vi "ActionVIOnDelete.vi"(6 "All deleted Refs":T1[](array[typedef]) format="%.0x", 8 "error in (no error)":errorcluster, 11 "Item Ref in":T1 format="%.0x") -> (0 "error out":errorcluster, 3 "Item Ref out":T1 format="%.0x")   [LabVIEW 2015, in "UDP-Custom-Device System Explorer.lvlib"]
uses:
  UDP-Custom-Device System Explorer.lvlib
  <vilib>/NI Veristand/Custom Device API/Custom Device Item Ref.ctl
  Shared/Constants.vi
  <vilib>/NI Veristand/Custom Device Tools/Custom Device Utility Library/NI VeriStand - Search for Item by GUID.vi
  <vilib>/NI VeriStand/Custom Device Tools/Custom Device Utility Library/Custom Device Utility Library.lvlib
  Shared/UDP-Custom-Device Shared.lvlib
  <vilib>/NI VeriStand/Custom Device API/Custom Device API.lvlib
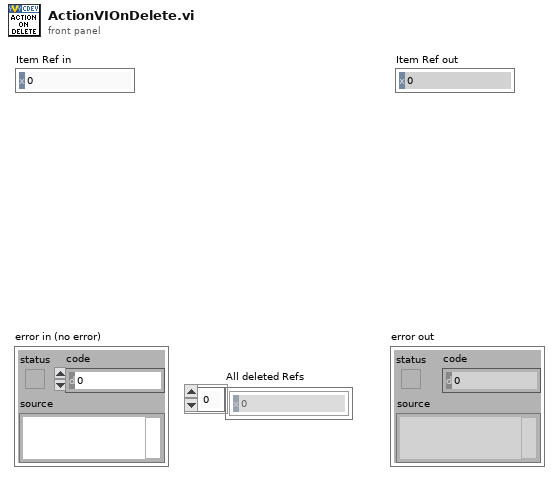
[diagram p1: front panel]
types:
  T1 = typedef "Custom Device API.lvlib/Custom Device Item Ref.ctl" = u64
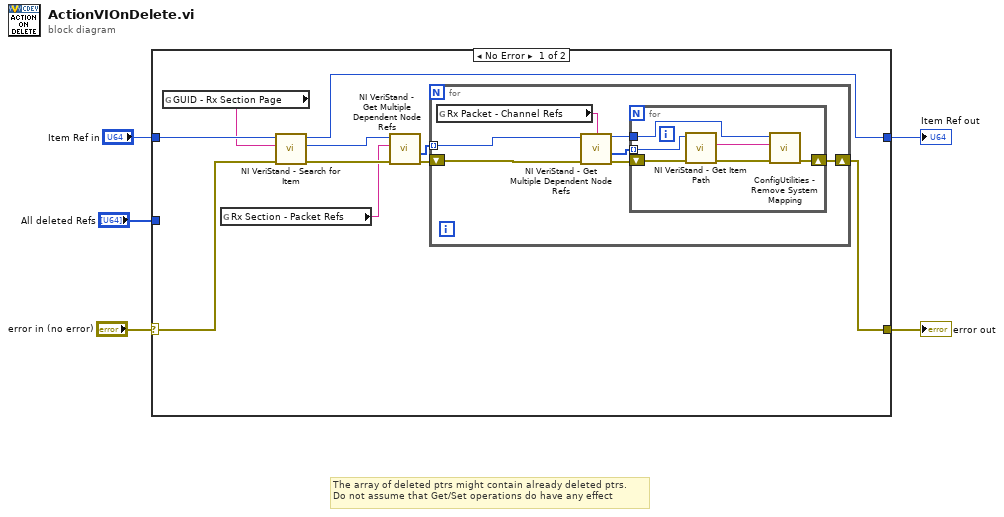
[diagram p0: block diagram]
diagram:
  # "The array of deleted ptrs might contain already deleted ptrs.\nDo not assume that Get/Set operations do have any effect"
  n1 = case shown="No Error" "error in (no error)" {
    selector: "error in (no error)" -> [w14 w30]
    tunnel: [w13 w30] -> w4
    tunnel: "Item Ref in" -> [w15 w29]
    tunnel: [w11 w29] -> w2
    tunnel: "All deleted Refs" -> [_ _]
    frame No Error {
      n2 = global read "Constants.vi" "GUID - Rx Section Page"() -> (w12:string)
      n3 = global read "Constants.vi" "Rx Section - Packet Refs"() -> (w8:string)
      n4 = call-poly <vilib>:"NI VeriStand - Search for Item.vi"("error in"=w14, "Item GUID"=w12, "Section Ref in"=w15) -> ("error out"=w10:errorcluster, "Item Ref"=w9:T1, "Section Ref out"=w11:T1)  [unwired: 5 in, 1 out]
      n5 = call <vilib>:"NI VeriStand - Get Multiple Dependent Node Refs.vi"("error in (no error)"=w10, "Base Property Name"=w8, "Item Ref in"=w9) -> ("error out"=w7:errorcluster, "Dependent Node Refs"=w6:T1[])  [unwired: 6 in, 1 out]
      n6 = for {
        tunnel: w6 -> [w16] mode=indexing
        shift-right: [w19] -> w13
        shift-left: w7 -> [w22]
        n7 = global read "Constants.vi" "Rx Packet - Channel Refs"() -> (w21:string)
        n8 = call <vilib>:"NI VeriStand - Get Multiple Dependent Node Refs.vi"("error in (no error)"=w22, "Base Property Name"=w21, "Item Ref in"=w16) -> ("error out"=w20:errorcluster, "Dependent Node Refs"=w17:T1[], "Item Ref out"=w18:T1)  [unwired: 6 in]
        n9 = for {
          shift-right: [w28] -> w19
          shift-left: w20 -> [w25]
          tunnel: w18 -> [w23]
          tunnel: w17 -> [w24] mode=indexing
          n10 = call <vilib>:"NI VeriStand - Get Item Path.vi"("error in (no error)"=w25, "Item Ref in"=w24) -> ("error out"=w27:errorcluster, "Path"=w26:string)  [unwired: 6 in, 2 out]
          n11 = call "ConfigUtilities - Remove System Mapping.vi"("error in (no error)"=w27, "Channel Path Destination"=w26, "Item Ref in"=w23) -> ("error out"=w28:errorcluster)  [unwired: 7 in, 1 out]
        }
      }
    }
    frame Error {
    }
  }
  "error out" <- w4
  "Item Ref out" <- w2
